vi "Write Cooler Enqueuer.vi"(10 "Cooler Enqueuer":refnum<class "Message Enqueuer.lvclass">, 11 "Cooler Controller in":refnum<class "Cooler Controller.lvclass">) -> (3 "Cooler Controller out":refnum<class "Cooler Controller.lvclass">)   [LabVIEW 2025, in "Cooler Controller.lvlib" / "Cooler Controller.lvclass"]
doc: "This VI tells the controller what cooler it is controlling. You may pass a Not A Refnum enqueuer as input to indicate that the controller is not in control of any cooler."
uses:
  Cooler Controller.lvclass
  <vilib>/ActorFramework/Message Enqueuer/Message Enqueuer.lvclass
  Cooler Controller.lvclass/Cooler Controller.ctl
  Level Controller/Level Controller/Deadband.ctl
  Level Controller/Write Deadband Msg/Write Deadband Msg.lvclass/Write Deadband Msg.ctl
  <vilib>/ActorFramework/Message Enqueuer/Message Enqueuer.lvclass/Message Enqueuer.ctl
  <vilib>/ActorFramework/Message Enqueuer/Enqueue.vi
  Level Controller/Write Deadband Msg/Write Deadband Msg.lvclass
  C:/Program Files/National Instruments/LabVIEW 2025/vi.lib/ActorFramework/Message/Message.lvclass
  <vilib>/ActorFramework/Message Priority Queue/Priority Enqueue.vi
  Level Controller/Level Controller/Level Controller.lvclass
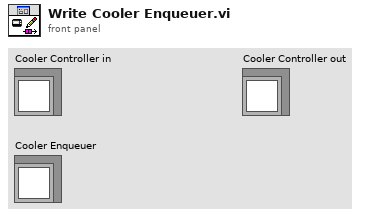
[diagram p1: front panel]
types:
  T1 = typedef "Level Controller.lvlib/Level Controller.lvclass/Deadband.ctl" = cluster{"Low":dbl, "High":dbl}
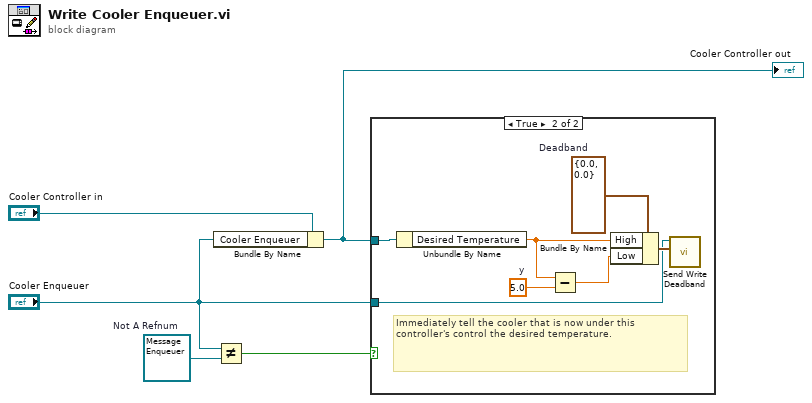
[diagram p0: block diagram]
diagram:
  w4 = refnum<class "Message Enqueuer.lvclass"> refnum  # Not A Refnum
  n1 = Bundle By Name(cluster="Cooler Controller in", "Cooler Enqueuer"="Cooler Enqueuer") -> (w2:refnum<class "Cooler Controller.lvclass">)
  "Cooler Controller out" <- w2
  n2 = Not Equal?(x="Cooler Enqueuer", y=w4) -> (x != y?=w3:bool)
  n3 = case shown="True" w3 {
    tunnel: w2 -> [_ w12]
    tunnel: "Cooler Enqueuer" -> [_ w6]
    frame False {
    }
    frame True {
      w10 = 5.0  # y
      w11 = T1 {"Low"=0.0, "High"=0.0}  # Deadband
      # "Immediately tell the cooler that is now under this controller's control the desired temperature."
      n4 = Unbundle By Name(w12) -> ("Desired Temperature"=w9:dbl)
      n5 = Subtract(x=w9, y=w10) -> (x-y=w8:dbl)
      n6 = Bundle By Name(cluster=w11, "High"=w9, "Low"=w8) -> (w7:T1)
      n7 = call "Send Write Deadband.vi"("Deadband"=w7, "Message Enqueuer"=w6) -> ()  [unwired: 9 in, 1 out]
    }
  }
